vi "Wavelet Packet - Join Node.vi"() -> ()   [LabVIEW 2023]
doc: "This example shows how to join a non-terminal wavelet packet node specified by the node path with the WA WP Joint VI. You cannot perform node-joining operations on terminal nodes.\n\n<b>Instructions:</b>\nRun this VI. Define the node to join."
uses:
  <vilib>/addons/Wavelet Analysis/typedefs.llb/WA Data.ctl
  <vilib>/addons/Wavelet Analysis/wavelet packet.llb/WA WP Decomposition (Waveform).vi
  <vilib>/addons/_Advanced Signal Processing/NI_AdvSigProcWA.lvlib
panel:
  in  "stop":bool
  out "Wavelet Packet Tree":picture
  in  "Node to joint":string="001"
  # "Overview: Shows how to join a non-terminal wavelet packet node specified by the node path with the WA WP Joint VI. You cannot perform node-joining operations on terminal nodes.\nRequirements: LabVIEW Full Development System, Advanced Signal Processing Toolkit\nInstructions: \n1. Run this VI. Define the node to join.\n2. Click Stop to stop the VI."
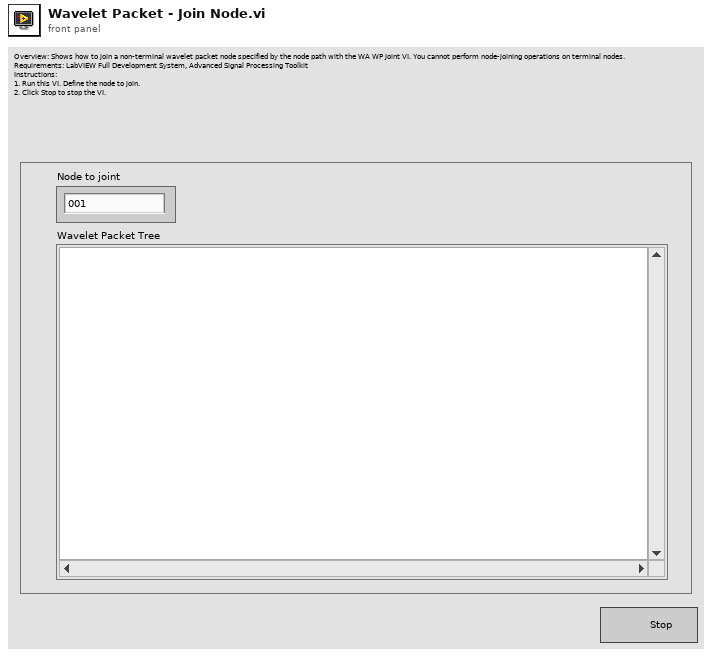
[diagram p1: front panel]
types:
  T1 = typedef "NI_AdvSigProcWA.lvlib/WA Data.ctl" = u16
  T2 = typedef "NI_AdvSigProcWA.lvlib/WA Generic Ref.ctl" = cluster{"ref":u64, "t0":timestamp, "dt":dbl}
  T3 = typedef "LVBoundsTypeDef.ctl" = cluster{"Width":u32, "Height":u32}
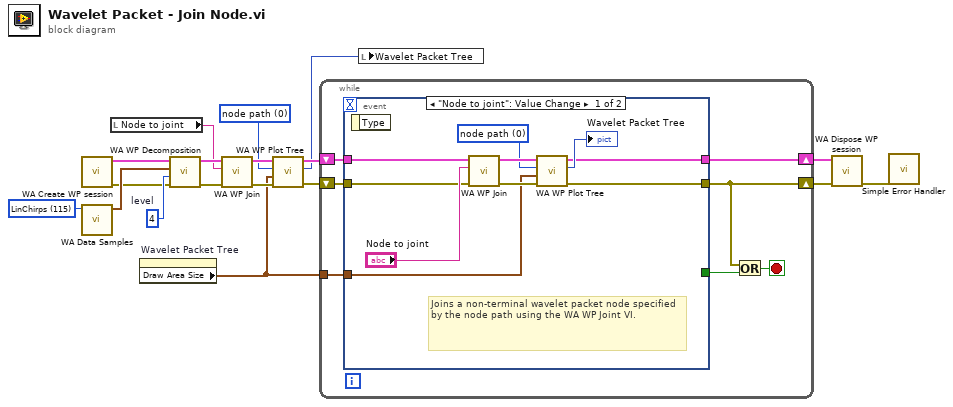
[diagram p0: block diagram]
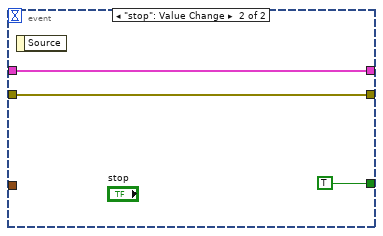
[diagram p2: hidden frame]
diagram:
  w4 = T1 115 items=["1D Example Data"=100, "-"=101, "Doppler"=102, "HOP"=103, "TF Sine"=104, "Noisy Doppler"=105, "Sea Temperature"=106, "Sp500"=107, "Power Line"=108, "Engine Knocking"=109, "HeaviSine"=110, "Bumps"=111, "Blocks"=112, "Piece Regular"=113, "HypChirps"=114, "LinChirps"=115, "Chirps"=116, "Piece Polynomial"=117, "ECG"=131, "-"=118, "2D Example Data"=119, "-"=120, "Finger Print (Image)"=121, "Iris Flower (Image)"=122, "Mammogram (Image)"=123, "Lake (Image)"=127, "Two Can 1 (Image)"=132, "Two Can 2 (Image)"=133, "Camera Man (Image)"=134] ("data")
  w6 = u16 0 items=["node path", "(depth, pos)", "entropy"] ("display mode")
  w18 = 4  # level
  n1 = call <vilib>:"WA Create WP session.vi"() -> ("error out"=w16:errorcluster, "WP session out"=w15:T2)  [unwired: 1 in, 9 out]
  n2 = call <vilib>:"WA Data Samples.vi"("data"=w4) -> ("signal"=w17:waveform(dbl))  [unwired: 10 out]
  n3 = local read "Node to joint"() -> (w10:string)
  n4 = property on="Wavelet Packet Tree" class="Pict"() -> ("Draw Area Size"=w7:T3)  [unwired: 2 in, 2 out]
  n5 = call-poly <vilib>:"WA WP Decomposition.vi"("error in (no error)"=w16, "levels"=w18, "signal"=w17, "WP session"=w15) -> ("error out"=w13:errorcluster, "WP session out"=w14:T2)  [unwired: 1 in, 5 out]
  n6 = call <vilib>:"WA WP Join.vi"("error in (no error)"=w13, "path"=w10, "WP session"=w14) -> ("error out"=w11:errorcluster, "WP session out"=w12:T2)  [unwired: 1 in, 6 out]
  n7 = call <vilib>:"WA WP Plot Tree.vi"("error in (no error)"=w11, "draw area size"=w7, "display mode"=w6, "WP session"=w12) -> ("error out"=w8:errorcluster, "tree plot"=w5:picture, "WP session out"=w9:T2)  [unwired: 5 out]
  n8 = while {
    tunnel: w7 -> [w23]
    shift-right: [w20] -> w1
    shift-left: w9 -> [w25]
    shift-right: [w19] -> w2
    shift-left: w8 -> [w24]
    stop <- w21 stop-if-true
    n9 = event shown="[0] \"Node to joint\": Value Change" {
      selector: _ -> [_ _]
      dyn-events: _ -> [_ _]
      timeout: _ -> [_ _]
      tunnel: [w31 w37] -> w20
      tunnel: w25 -> [w30 w37]
      tunnel: w24 -> [w29 w36]
      tunnel: w23 -> [w27 _]
      tunnel: [_ TRUE] -> w22
      tunnel: [w26 w36] -> w19
      event "Node to joint": Value Change {
        w32 = u16 0 items=["node path", "(depth, pos)", "entropy"] ("display mode")
        # "Joins a non-terminal wavelet packet node specified by the node path using the WA WP Joint VI."
        n10 = event-data() -> ()  [unwired: 2 out]
        n11 = call <vilib>:"WA WP Join.vi"("error in (no error)"=w29, "path"="Node to joint", "WP session"=w30) -> ("error out"=w28:errorcluster, "WP session out"=w35:T2)  [unwired: 1 in, 6 out]
        n12 = call <vilib>:"WA WP Plot Tree.vi"("error in (no error)"=w28, "draw area size"=w27, "display mode"=w32, "WP session"=w35) -> ("error out"=w26:errorcluster, "tree plot"=→"Wavelet Packet Tree":picture, "WP session out"=w31:T2)  [unwired: 5 out]
      }
      event "stop": Value Change {
        n13 = event-data() -> ()  [unwired: 2 out]
      }
    }
    n14 = Or(x=w19, y=w22) -> (x .or. y?=w21:bool)
  }
  n15 = local write "Wavelet Packet Tree"(w5) -> ()
  n16 = call <vilib>:"WA Dispose WP session.vi"("error in (no error)"=w2, "WP session"=w1) -> ("error out"=w3:errorcluster)  [unwired: 9 out]
  n17 = call <vilib>:"Simple Error Handler.vi"("error in (no error)"=w3) -> ()  [unwired: 1 in, 8 out]
